vi "Write Logs.vi"(7 "Prepend timestamp":bool, 10 "Log entries":string[](array[string]), 11 "SolutionBuilder in":refnum<class "SolutionBuilder.lvclass">) -> (3 "SolutionBuilder out":refnum<class "SolutionBuilder.lvclass">)   [LabVIEW 2019, in "SolutionBuilder.lvlib" / "SolutionBuilder.lvclass"]
uses:
  SolutionBuilder.lvclass
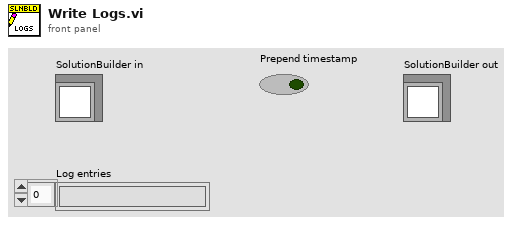
[diagram p1: front panel]
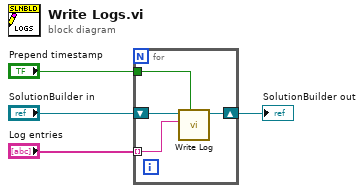
[diagram p0: block diagram]
diagram:
  n1 = for {
    tunnel: "Prepend timestamp" -> [w6]
    shift-right: [w7] -> w3
    shift-left: "SolutionBuilder in" -> [w8]
    tunnel: "Log entries" -> [w5] mode=indexing
    n2 = call-dynamic "Write Log.vi"("Prepend timestamp"=w6, "Log entry"=w5, "SolutionBuilder in"=w8) -> ("SolutionBuilder out"=w7:refnum<class "SolutionBuilder.lvclass">)  [unwired: 8 in]
  }
  "SolutionBuilder out" <- w3
